vi "Check Bench File Match Config File.vi"(0 "Bench File Test Number":string[](array[string]), 5 "Config File Test Number":string[](array[string]), 7 "Bench File Test Name":string[](array[string]), 9 "Config File Test Name":string[](array[string]), 11 "error in":errorcluster, 12 "Bench File Test Unit":string[](array[string]), 13 "Config File Test Unit":string[](array[string])) -> (15 "error out":errorcluster)   [LabVIEW 2020, in "GUCalibration2.lvlib"]
uses:
  GUCalibration2.lvlib
  Controls/Error Enum.ctl
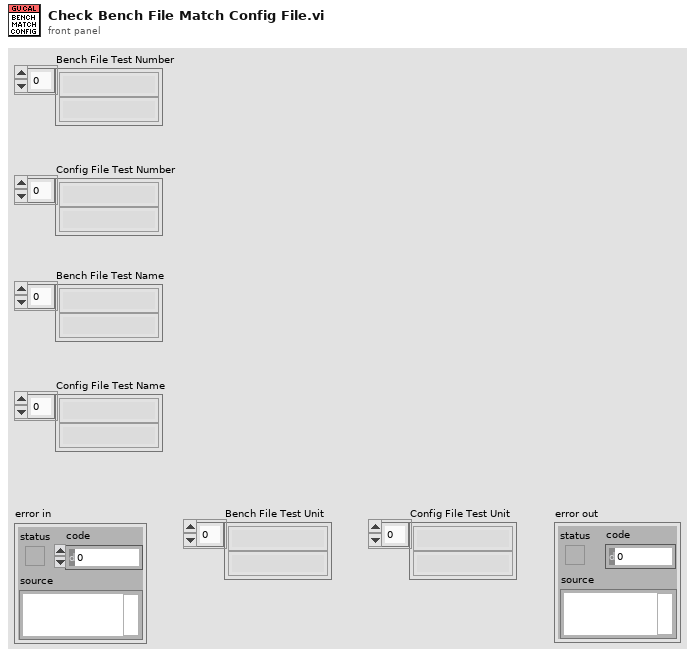
[diagram p1: front panel]
types:
  T1 = typedef "GUCalibration2.lvlib/Error Enum.ctl" = enum16{"Error Template Case", "Duplicated GU Number", "Test Items Mismatch"}
  T2 = cluster{i32, "trimmed string":string, "trimmed string":string}
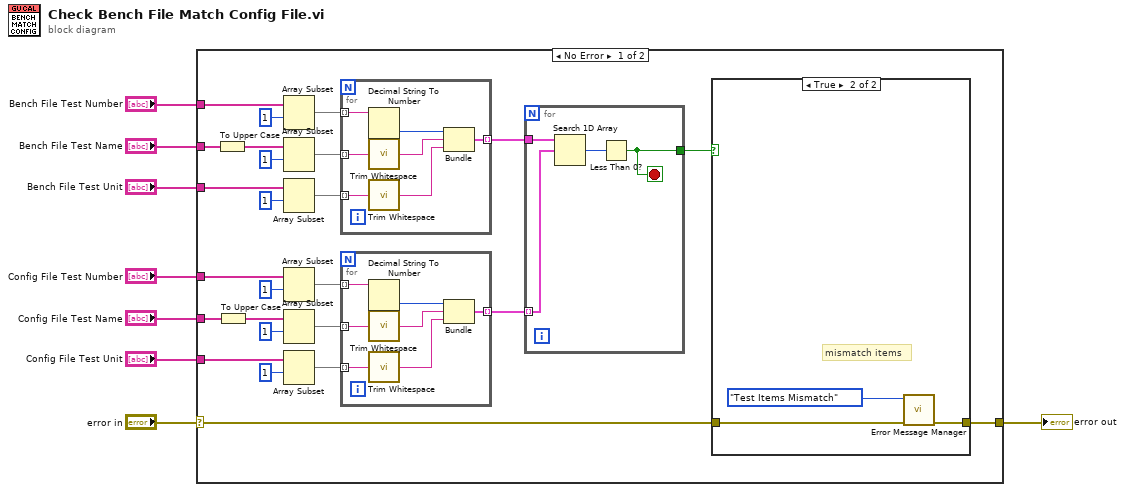
[diagram p0: block diagram]
diagram:
  n1 = case shown="No Error" "error in" {
    selector: "error in" -> [w32 w56]
    tunnel: "Bench File Test Number" -> [w31 _]
    tunnel: "Config File Test Number" -> [w28 _]
    tunnel: [w33 w56] -> w6
    tunnel: "Bench File Test Name" -> [w25 _]
    tunnel: "Config File Test Name" -> [w24 _]
    tunnel: "Bench File Test Unit" -> [w18 _]
    tunnel: "Config File Test Unit" -> [w21 _]
    frame No Error {
      n2 = To Upper Case(1:w25) -> (0:w23:string[])
      n3 = To Upper Case(1:w24) -> (0:w22:string[])
      n4 = Array Subset(array=w31, index=1) -> (w17:string[])  [unwired: 1 in]
      n5 = Array Subset(array=w23, index=1) -> (w16:string[])  [unwired: 1 in]
      n6 = Array Subset(array=w18, index=1) -> (w15:string[])  [unwired: 1 in]
      n7 = Array Subset(array=w28, index=1) -> (w14:string[])  [unwired: 1 in]
      n8 = Array Subset(array=w22, index=1) -> (w13:string[])  [unwired: 1 in]
      n9 = Array Subset(array=w21, index=1) -> (w12:string[])  [unwired: 1 in]
      n10 = for {
        tunnel: w17 -> [w51] mode=indexing
        tunnel: w16 -> [w50] mode=indexing
        tunnel: [w47] -> w11 mode=indexing
        tunnel: w15 -> [w46] mode=indexing
        n11 = Decimal String To Number(string=w51) -> (number=w49:i32)  [unwired: 2 in, 1 out]
        n12 = call <vilib>:"Trim Whitespace.vi"("string"=w50) -> ("trimmed string"=w48:string)  [unwired: 1 in]
        n13 = call <vilib>:"Trim Whitespace.vi"("string"=w46) -> ("trimmed string"=w45:string)  [unwired: 1 in]
        n14 = Bundle(w49, "trimmed string"=w48, "trimmed string"=w45) -> (w47:T2)  [unwired: 1 in]
      }
      n15 = for {
        tunnel: [w42] -> w10 mode=indexing
        tunnel: w14 -> [w40] mode=indexing
        tunnel: w13 -> [w39] mode=indexing
        tunnel: w12 -> [w38] mode=indexing
        n16 = Decimal String To Number(string=w40) -> (number=w44:i32)  [unwired: 2 in, 1 out]
        n17 = call <vilib>:"Trim Whitespace.vi"("string"=w39) -> ("trimmed string"=w43:string)  [unwired: 1 in]
        n18 = call <vilib>:"Trim Whitespace.vi"("string"=w38) -> ("trimmed string"=w41:string)  [unwired: 1 in]
        n19 = Bundle(w44, "trimmed string"=w43, "trimmed string"=w41) -> (w42:T2)  [unwired: 1 in]
      }
      n20 = for {
        tunnel: w11 -> [w37]
        tunnel: w10 -> [w36] mode=indexing
        tunnel: [w34] -> w9
        stop <- w34 stop-if-true
        n21 = Search 1D Array(1D array=w37, element=w36) -> (index of element=w35:i32)  [unwired: 1 in]
        n22 = Less Than 0?(x=w35) -> (x < 0?=w34:bool)
      }
      n23 = case shown="True" w9 {
        tunnel: w32 -> [w52 w55]
        tunnel: [w52 w54] -> w33
        frame False {
        }
        frame True {
          # "mismatch items"
          n24 = call "Error Message Manager.vi"("error in"=w55, "Error Selection"=Error_Enum."Test Items Mismatch") -> ("error out"=w54:errorcluster)  [unwired: 9 in]
        }
      }
    }
    frame Error {
    }
  }
  "error out" <- w6
